vi "Get_Sweep_Speed_table.vi"(8 "error in (no error)":errorcluster, 11 ".NET Reference in":refnum<k24>) -> (0 "error out":errorcluster, 2 "Get_Sweep_Speed_table":dbl[](array[numeric]), 3 "Reference out":refnum<k24>)   [LabVIEW 2017]
uses:
  D:/test/ILSTS/LV_IL/LV_IL_Sample_x64/DLL/InstrumentDLL.dll
  DLL/InstrumentDLL.dll
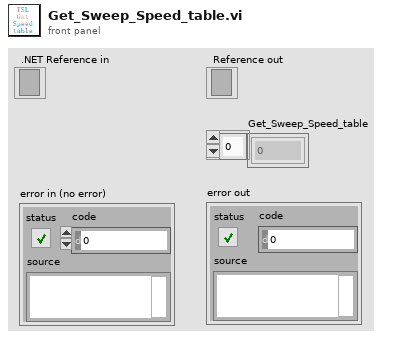
[diagram p1: front panel]
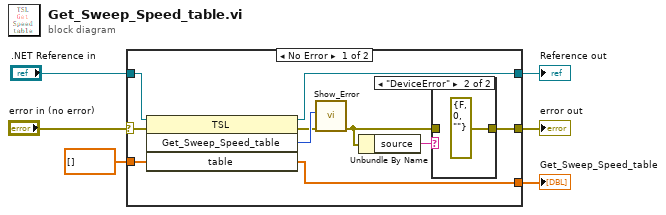
[diagram p0: block diagram]
diagram:
  n1 = case shown="No Error" "error in (no error)" {
    selector: "error in (no error)" -> [w12 w21]
    tunnel: [w16 w19] -> w6
    tunnel: [w7 w21] -> w5
    tunnel: dbl[] [] ("table") -> [w15 w19]
    tunnel: ".NET Reference in" -> [w11 w20]
    tunnel: [w10 w20] -> w1
    frame No Error {
      n2 = invoke on="调用节点" class="TSL" method="Get_Sweep_Speed_table"(reference=w11, error in=w12, "table"=w15) -> (reference out=w10:refnum<k24>, error out=w13:errorcluster, "Get_Sweep_Speed_table"=w14:i32, "table"=w16:dbl[])  [unwired: 1 in]
      n3 = call "Show_Error.vi"("error in (no error)"=w13, "Error"=w14) -> ("error out"=w8:errorcluster)  [unwired: 9 in]
      n4 = Unbundle By Name(w8) -> ("source"=w9:string)
      n5 = case shown="\"DeviceError\"" w9 {
        tunnel: w8 -> [w17 _]
        tunnel: [w17 errorcluster {"status"=FALSE, "code"=0, "source"=""} ("error out")] -> w7
        frame "0", Default {
        }
        frame "DeviceError" {
        }
      }
    }
    frame Error {
    }
  }
  "Get_Sweep_Speed_table" <- w6
  "error out" <- w5
  "Reference out" <- w1
